vi "Server Restart Client.vi"() -> ()   [LabVIEW 2020, in "VectoScratch.lvlib"]
uses:
  VectoScratch.lvlib
  Vecto/LocalEventCollector/Event.ctl
  lv-volatus/Volatus/Event Level.ctl
  Vecto/Event Level.ctl
  Vecto/proto/TcpClientHello/Data.ctl
  Vecto/LocalEventCollector/LocalEventCollector.lvclass
  C:/dev/lv20CE/relink/lv-vecto/Vecto/EventLogHandler/EventLogHandler.lvclass
  Vecto/TCPMessaging/TCPMessaging.lvclass
  Vecto/SequenceCountService/SequenceCountService.lvclass
  Vecto/EventLoggingService/EventLoggingService.lvclass
  Vecto/Vecto.lvlib
  Vecto/proto/TcpClientHello/TcpClientHello.lvlib
  lv-volatus/Volatus/Volatus.lvlib
panel:
  out "error out":errorcluster
  out "Events":T1[](array[typedef])
  in  "Stop":bool
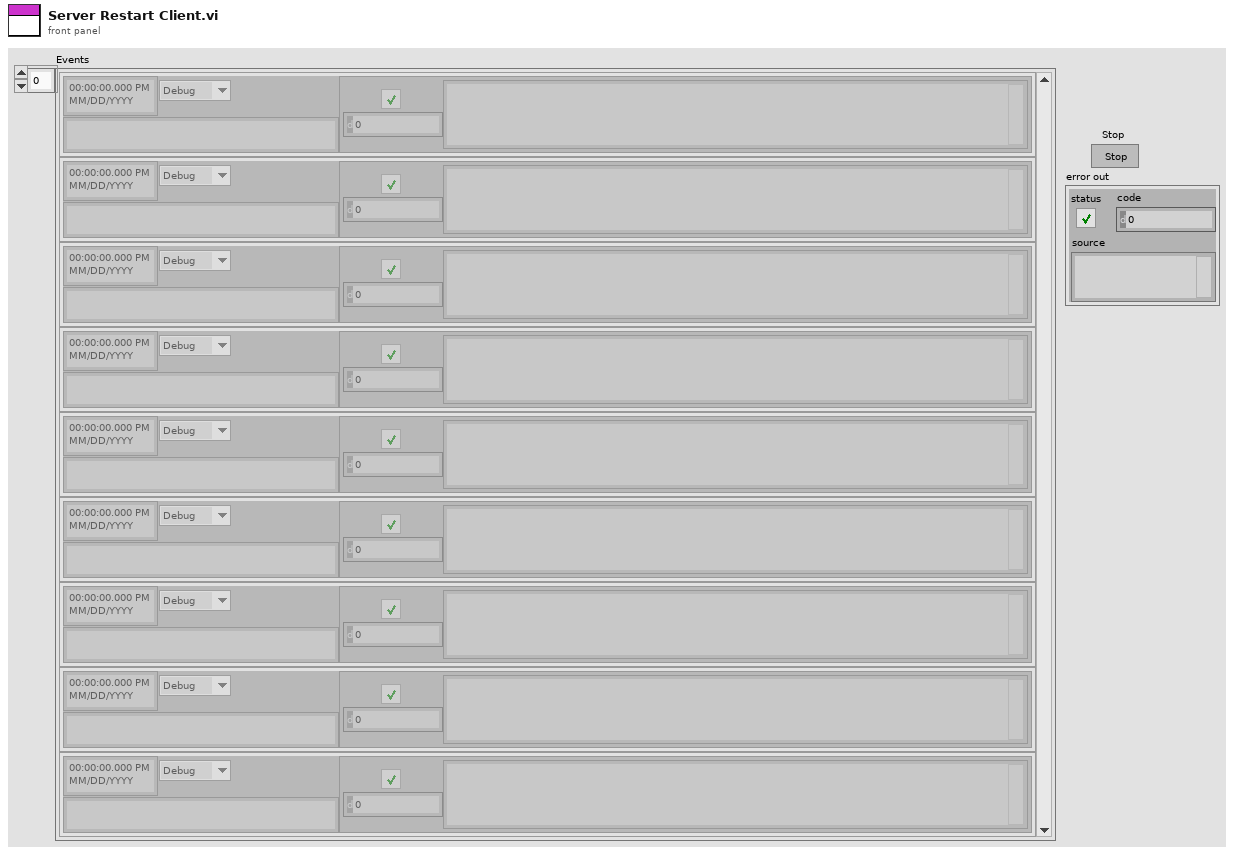
[diagram p1: front panel]
types:
  T1 = typedef "Vecto.lvlib/LocalEventCollector.lvclass/Event.ctl" = cluster{"Time Stamp":timestamp, "Event Level":T2, "Message":string, "Error":errorcluster}
  T2 = typedef "Volatus.lvlib/Event Level.ctl" = enum16{"Debug", "Info", "Warning", "Error"}
  T3 = typedef "TcpClientHello.lvlib/Data.ctl" = cluster{"node_id":u32, "system":string, "cluster":string, "node_name":string, "app_version":string, "config_version":string, "config_hash":string}
  T4 = typedef "Vecto.lvlib/Event Level.ctl" = enum16{"Debug", "Info", "Warning", "Error"}
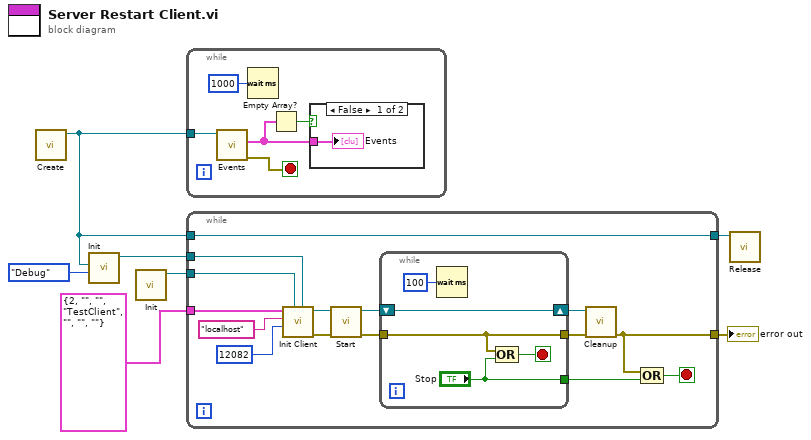
[diagram p0: block diagram]
diagram:
  n1 = call "Create.vi"() -> ("LocalEventCollector out"=w5:refnum<class "LocalEventCollector.lvclass">)  [unwired: 10 in, 1 out]
  n2 = call "Init.vi"("Minimum Event Level"=Event_Level."Debug", "EventLogger"=w5) -> ("EventLoggingService out"=w6:refnum<class "EventLoggingService.lvclass">)  [unwired: 8 in, 1 out]
  n3 = call "Init.vi"() -> ("SequenceCountService out"=w7:refnum<class "SequenceCountService.lvclass">)  [unwired: 10 in, 1 out]
  n4 = while {
    tunnel: w5 -> [w12]
    stop <- w11 stop-if-true
    n5 = call "Events.vi"("LocalEventCollector in"=w12) -> ("error out"=w11:errorcluster, "Events"=w9:T1[])  [unwired: 8 in, 1 out]
    n6 = Wait (ms)(milliseconds to wait=u32 1000) -> ()  [unwired: 1 out]
    n7 = Empty Array?(array=w9) -> (empty?=w8:bool)
    n8 = case shown="False" w8 {
      tunnel: w9 -> [w13 _]
      frame False {
        "Events" <- w13
      }
      frame True {
      }
    }
  }
  n9 = while {
    tunnel: w7 -> [w28]
    tunnel: w6 -> [w27]
    tunnel: [w20] -> w3
    tunnel: w5 -> [w17]
    tunnel: [w17] -> w4
    tunnel: T3 {"node_id"=2, "system"="", "cluster"="", "node_name"="TestClient", "app_version"="", "config_version"="", "config_hash"=""} ("Client Info") -> [w16]
    stop <- w18 stop-if-true
    n10 = call "Init Client.vi"("EventLogger"=w27, "SequenceCountService"=w28, "Remote Port"=u16 12082, "Remote Address"="localhost", "Client Info"=w16) -> ("error out"=w26:errorcluster, "TCPMessaging out"=w25:refnum<class "TCPMessaging.lvclass">)  [unwired: 5 in]
    n11 = call "Start.vi"("error in (no error)"=w26, "TCPMessaging in"=w25) -> ("error out"=w24:errorcluster, "TCPMessaging out"=w23:refnum<class "TCPMessaging.lvclass">)  [unwired: 8 in]
    n12 = while {
      tunnel: w24 -> [w30]
      shift-right: [w32] -> w21
      shift-left: w23 -> [w32]
      tunnel: [w30] -> w22
      tunnel: ["Stop"] -> w19
      stop <- w31 stop-if-true
      n13 = Wait (ms)(milliseconds to wait=u32 100) -> ()  [unwired: 1 out]
      n14 = Compound Arithmetic op=OR(w30, "Stop") -> (w31:bool)
    }
    n15 = call "Cleanup.vi"("error in (no error)"=w22, "TCPMessaging in"=w21) -> ("error out"=w20:errorcluster)  [unwired: 9 in]
    n16 = Compound Arithmetic op=OR(w20, w19) -> (w18:bool)
  }
  "error out" <- w3
  n17 = call "Release.vi"("LocalEventCollector in"=w4) -> ()  [unwired: 10 in, 1 out]
